vi "Loop_ACT_Drive.vi"() -> ()   [LabVIEW 2016, in "WC_Drive.lvlib"]
uses:
  WC_Drive.lvlib
  TypeDef/CLUSTER_Drive_HW_SRX_Status.ctl
  TypeDef/CLUSTER_4296_SRX_Status.ctl
  TypeDef/CLUSTER_SRX_Status Data.ctl
  TypeDef/CLUSTER_SRX_Encoder Data.ctl
  TypeDef/CLUSTER_SRX_PWM Data.ctl
  TypeDef/CLUSTER_SRX_Analog Data.ctl
  TypeDef/CLUSTER_SRX_Limit Switch Data.ctl
  TypeDef/CLUSTER_SRX_Profile Data.ctl
  TypeDef/ENUM_Drive_ACT Loop_Mode.ctl
  TypeDef/CLUSTER_Left and Right.ctl
  Globals/Global_STOP.vi
  Global_SM Write_Data Out.vi
  Global_ACT Write_Data Out.vi
panel:
  out "Right Data":dbl
  out "Left Data":dbl
  out "Cycle Time (S)":dbl format="%.3g"
  in  "Target Time(ms)":u32=50
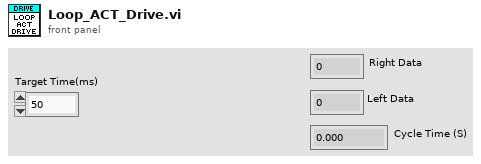
[diagram p1: front panel]
types:
  T1 = typedef "CLUSTER_Left and Right.ctl" = cluster{"Left":dbl, "Right":dbl}
  T2 = typedef "ENUM_Drive_ACT Loop_Mode.ctl" = enum16{"Stop", "VBus", "Profile"}
  T3 = typedef "CLUSTER_Drive_HW_SRX_Status.ctl" = cluster{"Rear Left":T4, "Rear Right":T4, "Front Left":T4, "Front Right":T4}
  T4 = typedef "CLUSTER_4296_SRX_Status.ctl" = cluster{"Status":T5, "Encoder":T6, "PWM ":T7, "Analog":T8, "Limit Switches":T9, "Profile":T10}
  T5 = typedef "CLUSTER_SRX_Status Data.ctl" = cluster{"Module Enabled":bool, "Current Profile Slot Select":dbl, "Brake is Enabled":bool, "Applied Throttle":dbl, "Current":dbl, "Battery Voltage":dbl, "Sticky Fault - Under Voltage":bool, "Temperature (C)":dbl, "Sticky Fault - Over Temp":bool, "CAN Error":errorcluster, "Control 5 Is Supported":bool}
  T6 = typedef "CLUSTER_SRX_Encoder Data.ctl" = cluster{"Closed Loop Error":dbl, "Sensor Position":dbl, "Sensor Velocity":dbl, "Encoder Position":dbl, "Encoder Velocity":dbl, "Encoder Index Count":dbl, "Encoder A Pin State":bool, "Encoder B Pin State":bool, "Encoder Index Pin State":bool, "Pos Div 8":bool, "Vel Div 4":bool}
  T7 = typedef "CLUSTER_SRX_PWM Data.ctl" = cluster{"Closed Loop Error":dbl, "Pulse Width Position":i32, "Pulse Width Velocity":i32, "Pulse Width Rise To Rise (us)":i32, "Pulse Width Rise To Fall (us)":i32}
  T8 = typedef "CLUSTER_SRX_Analog Data.ctl" = cluster{"Closed Loop Error":dbl, "Analog In":dbl, "Analog In Velocity":dbl}
  T9 = typedef "CLUSTER_SRX_Limit Switch Data.ctl" = cluster{"Forward Limit Switch Closed":bool, "Reverse Limit Switch Closed":bool, "Sticky Fault - Forward Limit":bool, "Sticky Fault - Reverse Limit":bool, "Sticky Fault - Forward Soft Limit":bool, "Sticky Fault - Reverse Soft Limit":bool}
  T10 = typedef "CLUSTER_SRX_Profile Data.ctl" = cluster{"Mot Prof Active Is Under Run":bool, "Mot Prof Active Has Under Run":bool, "Mot Prof Active Is Last":bool, "Mot Prof Active Velocity Only":bool, "Mot Prof Active Is Valid":bool, "Mot Prof Buffer Is Full":bool, "Mot Prof Active Profile Slot Select":i32, "Mot Prof NextID":i32, "Mot Prof Count":i32, "Mot Prof Active Velocity":dbl, "Mot Prof Active Position":dbl, "Mot Prof Output Enable":i32}
  T11 = typedef "WPI_RobotDriveDevRef.ctl" = cluster{"DevStatus":errorcluster, "Motors[]":T12[], "Square Inputs":bool, "Max Output":dbl}
  T12 = typedef "WPI_MotorControlDeviceRef.ctl" = cluster{"DeviceStatus":errorcluster, "Type":T13, "PWM":cluster{"PWM Channel":T14, "DeadBand":T15}, "CAN":cluster{"Device Number":u8, "SetOutput VI Ref":variant, "GetOutput VI Ref":variant, "Enable VI Ref":variant, "Disable VI Ref":variant, "Data":variant}, "Invert":bool}
  T13 = typedef "WPI_MotorControlType.ctl" = enum16{"PWM", "CAN"}
  T14 = typedef "FPGA_DIOPWMChannel.ctl" = enum8{"PWM 0", "PWM 1", "PWM 2", "PWM 3", "PWM 4", "PWM 5", "PWM 6", "PWM 7", "PWM 8", "PWM 9", "PWM MXP 0", "PWM MXP 1", "PWM MXP 2", "PWM MXP 3", "PWM MXP 4", "PWM MXP 5", "PWM MXP 6", "PWM MXP 7", "PWM MXP 8", "PWM MXP 9", "Invalid"}
  T15 = typedef "WPI_PWMDeadband.ctl" = cluster{"Name":string, "maxPositivePwm":i32, "minPositivePwm":i32, "centerPwm":i32, "maxNegativePwm":i32, "minNegativePwm":i32, "angularRange":u16}
  T16 = cluster{"RobotDriveDevRef":T11, "Target Time(ms)":u32, "Current Time":timestamp, "Previous Time":timestamp, "Cycle Time (S)":dbl, "SRX_Status":T3, "Mode":T2, "VBus":T1, "Cruise RPM":dbl, "MAX Velocity\n":dbl}
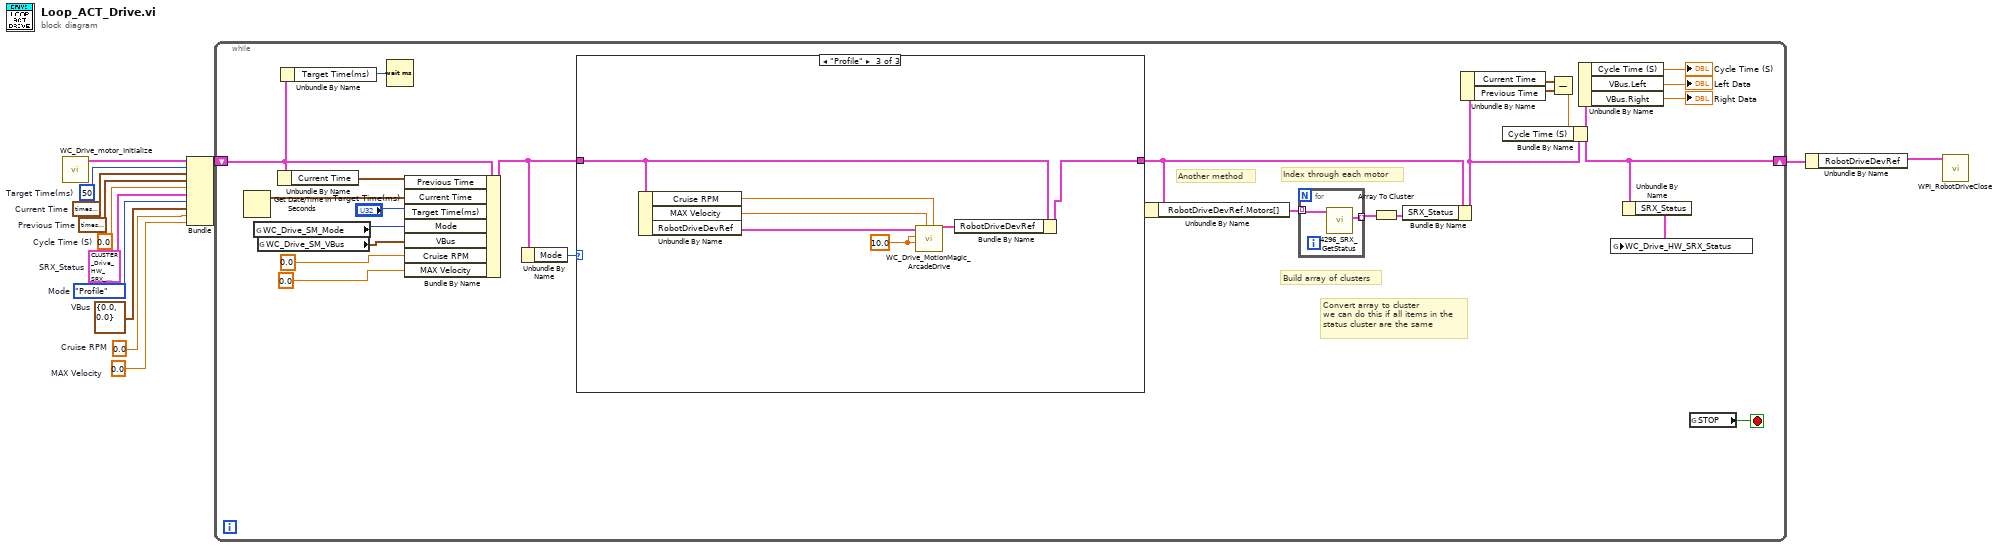
[diagram p0: block diagram]
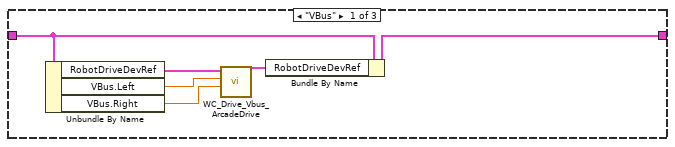
[diagram p2: hidden frame]
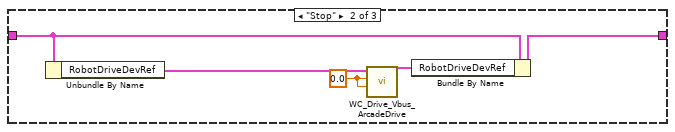
[diagram p3: hidden frame]
diagram:
  w1 = 0.0  # MAX Velocity
  w2 = 0.0  # Cruise RPM
  w3 = T1 {"Left"=0.0, "Right"=0.0}  # VBus
  w4 = ENUM_Drive_ACT_Loop_Mode."Profile"  # Mode
  w5 = T3 {"Rear Left"={"Status"={"Module Enabled"=FALSE, "Current Profile Slot Select"=0.0, "Brake is Enabled"=FALSE, "Applied Throttle"=0.0, "Current"=0.0, "Battery Voltage"=0.0, "Sticky Fault - Under Voltage"=FALSE, "Temperature (C)"=0.0, "Sticky Fault - Over Temp"=FALSE, "CAN Error"={"status"=FALSE, "code"=0, "source"=""}, "Control 5 Is Supported"=FALSE}, "Encoder"={"Closed Loop Error"=0.0, "Sensor Position"=0.0, "Sensor Velocity"=0.0, "Encoder Position"=0.0, "Encoder Velocity"=0.0, "Encoder Index Count"=0.0, "Encoder A Pin State"=FALSE, "Encoder B Pin State"=FALSE, "Encoder Index Pin State"=FALSE, "Pos Div 8"=FALSE, "Vel Div 4"=FALSE}, "PWM "={"Closed Loop Error"=0.0, "Pulse Width Position"=0, "Pulse Width Velocity"=0, "Pulse Width Rise To Rise (us)"=0, "Pulse Width Rise To Fall (us)"=0}, "Analog"={"Closed Loop Error"=0.0, "Analog In"=0.0, "Analog In Velocity"=0.0}, "Limit Switches"={"Forward Limit Switch Closed"=FALSE, "Reverse Limit Switch Closed"=FALSE, "Sticky Fault - Forward Limit"=FALSE, "Sticky Fault - Reverse Limit"=FALSE, "Sticky Fault - Forward Soft Limit"=FALSE, "Sticky Fault - Reverse Soft Limit"=FALSE}, "Profile"={"Mot Prof Active Is Under Run"=FALSE, "Mot Prof Active Has Under Run"=FALSE, "Mot Prof Active Is Last"=FALSE, "Mot Prof Active Velocity Only"=FALSE, "Mot Prof Active Is Valid"=FALSE, "Mot Prof Buffer Is Full"=FALSE, "Mot Prof Active Profile Slot Select"=0, "Mot Prof NextID"=0, "Mot Prof Count"=0, "Mot Prof Active Velocity"=0.0, "Mot Prof Active Position"=0.0, "Mot Prof Output Enable"=0}}, "Rear Right"={"Status"={"Module Enabled"=FALSE, "Current Profile Slot Select"=0.0, "Brake is Enabled"=FALSE, "Applied Throttle"=0.0, "Current"=0.0, "Battery Voltage"=0.0, "Sticky Fault - Under Voltage"=FALSE, "Temperature (C)"=0.0, "Sticky Fault - Over Temp"=FALSE, "CAN Error"={"status"=FALSE, "code"=0, "source"=""}, "Control 5 Is Supported"=FALSE}, "Encoder"={"Closed Loop Error"=0.0, "Sensor Position"=0.0, "Sensor Velocity"=0.0, "Encoder Position"=0.0, "Encoder Velocity"=0.0, "Encoder Index Count"=0.0, "Encoder A Pin State"=FALSE, "Encoder B Pin State"=FALSE, "Encoder Index Pin State"=FALSE, "Pos Div 8"=FALSE, "Vel Div 4"=FALSE}, "PWM "={"Closed Loop Error"=0.0, "Pulse Width Position"=0, "Pulse Width Velocity"=0, "Pulse Width Rise To Rise (us)"=0, "Pulse Width Rise To Fall (us)"=0}, "Analog"={"Closed Loop Error"=0.0, "Analog In"=0.0, "Analog In Velocity"=0.0}, "Limit Switches"={"Forward Limit Switch Closed"=FALSE, "Reverse Limit Switch Closed"=FALSE, "Sticky Fault - Forward Limit"=FALSE, "Sticky Fault - Reverse Limit"=FALSE, "Sticky Fault - Forward Soft Limit"=FALSE, "Sticky Fault - Reverse Soft Limit"=FALSE}, "Profile"={"Mot Prof Active Is Under Run"=FALSE, "Mot Prof Active Has Under Run"=FALSE, "Mot Prof Active Is Last"=FALSE, "Mot Prof Active Velocity Only"=FALSE, "Mot Prof Active Is Valid"=FALSE, "Mot Prof Buffer Is Full"=FALSE, "Mot Prof Active Profile Slot Select"=0, "Mot Prof NextID"=0, "Mot Prof Count"=0, "Mot Prof Active Velocity"=0.0, "Mot Prof Active Position"=0.0, "Mot Prof Output Enable"=0}}, "Front Left"={"Status"={"Module Enabled"=FALSE, "Current Profile Slot Select"=0.0, "Brake is Enabled"=FALSE, "Applied Throttle"=0.0, "Current"=0.0, "Battery Voltage"=0.0, "Sticky Fault - Under Voltage"=FALSE, "Temperature (C)"=0.0, "Sticky Fault - Over Temp"=FALSE, "CAN Error"={"status"=FALSE, "code"=0, "source"=""}, "Control 5 Is Supported"=FALSE}, "Encoder"={"Closed Loop Error"=0.0, "Sensor Position"=0.0, "Sensor Velocity"=0.0, "Encoder Position"=0.0, "Encoder Velocity"=0.0, "Encoder Index Count"=0.0, "Encoder A Pin State"=FALSE, "Encoder B Pin State"=FALSE, "Encoder Index Pin State"=FALSE, "Pos Div 8"=FALSE, "Vel Div 4"=FALSE}, "PWM "={"Closed Loop Error"=0.0, "Pulse Width Position"=0, "Pulse Width Velocity"=0, "Pulse Width Rise To Rise (us)"=0, "Pulse Width Rise To Fall (us)"=0}, "Analog"={"Closed Loop Error"=0.0, "Analog In"=0.0, "Analog In Velocity"=0.0}, "Limit Switches"={"Forward Limit Switch Closed"=FALSE, "Reverse Limit Switch Closed"=FALSE, "Sticky Fault - Forward Limit"=FALSE, "Sticky Fault - Reverse Limit"=FALSE, "Sticky Fault - Forward Soft Limit"=FALSE, "Sticky Fault - Reverse Soft Limit"=FALSE}, "Profile"={"Mot Prof Active Is Under Run"=FALSE, "Mot Prof Active Has Under Run"=FALSE, "Mot Prof Active Is Last"=FALSE, "Mot Prof Active Velocity Only"=FALSE, "Mot Prof Active Is Valid"=FALSE, "Mot Prof Buffer Is Full"=FALSE, "Mot Prof Active Profile Slot Select"=0, "Mot Prof NextID"=0, "Mot Prof Count"=0, "Mot Prof Active Velocity"=0.0, "Mot Prof Active Position"=0.0, "Mot Prof Output Enable"=0}}, "Front Right"={"Status"={"Module Enabled"=FALSE, "Current Profile Slot Select"=0.0, "Brake is Enabled"=FALSE, "Applied Throttle"=0.0, "Current"=0.0, "Battery Voltage"=0.0, "Sticky Fault - Under Voltage"=FALSE, "Temperature (C)"=0.0, "Sticky Fault - Over Temp"=FALSE, "CAN Error"={"status"=FALSE, "code"=0, "source"=""}, "Control 5 Is Supported"=FALSE}, "Encoder"={"Closed Loop Error"=0.0, "Sensor Position"=0.0, "Sensor Velocity"=0.0, "Encoder Position"=0.0, "Encoder Velocity"=0.0, "Encoder Index Count"=0.0, "Encoder A Pin State"=FALSE, "Encoder B Pin State"=FALSE, "Encoder Index Pin State"=FALSE, "Pos Div 8"=FALSE, "Vel Div 4"=FALSE}, "PWM "={"Closed Loop Error"=0.0, "Pulse Width Position"=0, "Pulse Width Velocity"=0, "Pulse Width Rise To Rise (us)"=0, "Pulse Width Rise To Fall (us)"=0}, "Analog"={"Closed Loop Error"=0.0, "Analog In"=0.0, "Analog In Velocity"=0.0}, "Limit Switches"={"Forward Limit Switch Closed"=FALSE, "Reverse Limit Switch Closed"=FALSE, "Sticky Fault - Forward Limit"=FALSE, "Sticky Fault - Reverse Limit"=FALSE, "Sticky Fault - Forward Soft Limit"=FALSE, "Sticky Fault - Reverse Soft Limit"=FALSE}, "Profile"={"Mot Prof Active Is Under Run"=FALSE, "Mot Prof Active Has Under Run"=FALSE, "Mot Prof Active Is Last"=FALSE, "Mot Prof Active Velocity Only"=FALSE, "Mot Prof Active Is Valid"=FALSE, "Mot Prof Buffer Is Full"=FALSE, "Mot Prof Active Profile Slot Select"=0, "Mot Prof NextID"=0, "Mot Prof Count"=0, "Mot Prof Active Velocity"=0.0, "Mot Prof Active Position"=0.0, "Mot Prof Output Enable"=0}}}  # SRX_Status
  w8 = 0.0  # Cycle Time (S)
  w13 = timestamp(0 s since 1904-01-01)  # Previous Time
  w12 = timestamp(0 s since 1904-01-01)  # Current Time
  w11 = u32 50  # Target Time(ms)
  n1 = call "WC_Drive_motor_Initialize.vi"() -> ("RobotDriveDevRef"=w7:T11)  [unwired: 11 in]
  n2 = Bundle("RobotDriveDevRef"=w7, "Target Time(ms)"=w11, "Current Time"=w12, "Previous Time"=w13, "Cycle Time (S)"=w8, "SRX_Status"=w5, "Mode"=w4, "VBus"=w3, "Cruise RPM"=w2, "MAX Velocity"=w1) -> (w10:T16)  [unwired: 1 in]
  n3 = while {
    shift-right: [w23] -> w9
    shift-left: w10 -> [w20]
    stop <- w38 stop-if-true
    # "Build array of clusters"
    # "Convert array to cluster\nwe can do this if all items in the\nstatus cluster are the same"
    # "Index through each motor"
    # "Another method"
    n4 = Get Date/Time In Seconds() -> (seconds since 1Jan1904=w37:timestamp)
    n5 = global read "Global_SM Write_Data Out.vi" "WC_Drive_SM_Mode"() -> (w27:T2)
    n6 = global read "Global_SM Write_Data Out.vi" "WC_Drive_SM_VBus"() -> (w16:T1)
    n7 = Unbundle By Name(w20) -> ("Current Time"=w36:timestamp)
    n8 = Unbundle By Name(w20) -> ("Target Time(ms)"=w32:u32)
    n9 = Wait (ms)(milliseconds to wait=w32) -> ()  [unwired: 1 out]
    n10 = Bundle By Name(cluster=w20, "Previous Time"=w36, "Current Time"=w37, "Target Time(ms)"="Target Time(ms)", "Mode"=w27, "VBus"=w16, "Cruise RPM"=0.0, "MAX Velocity"=0.0) -> (w26:T16)
    n11 = Unbundle By Name(w26) -> ("Mode"=w25:T2)
    n12 = case shown="\"Profile\"" w25 {
      tunnel: w26 -> [w42 w50 w54]
      tunnel: [w41 w49 w55] -> w21
      frame "VBus" {
        n13 = Unbundle By Name(w42) -> ("RobotDriveDevRef"=w46:T11, "VBus.Left"=w45:dbl, "VBus.Right"=w44:dbl)
        n14 = call "WC_Drive_Vbus_ArcadeDrive.vi"("Right Value"=w44, "Left Value"=w45, "RobotDriveDevRef"=w46) -> ("RobotDriveDevRef Out"=w43:T11)  [unwired: 7 in, 1 out]
        n15 = Bundle By Name(cluster=w42, "RobotDriveDevRef"=w43) -> (w41:T16)
      }
      frame "Stop" {
        w48 = 0.0 ("X axis value")
        n16 = Unbundle By Name(w50) -> ("RobotDriveDevRef"=w47:T11)
        n17 = call "WC_Drive_Vbus_ArcadeDrive.vi"("Right Value"=w48, "Left Value"=w48, "RobotDriveDevRef"=w47) -> ("RobotDriveDevRef Out"=w51:T11)  [unwired: 7 in, 1 out]
        n18 = Bundle By Name(cluster=w50, "RobotDriveDevRef"=w51) -> (w49:T16)
      }
      frame "Profile" {
        w57 = 10.0 ("X axis value")
        n19 = Unbundle By Name(w54) -> ("Cruise RPM"=w53:dbl, "MAX Velocity"=w52:dbl, "RobotDriveDevRef"=w58:T11)
        n20 = call "WC_Drive_MotionMagic_ArcadeDrive.vi"("Cruise RPM"=w53, "Max Velocity"=w52, "Right Value"=w57, "Left Value"=w57, "RobotDriveDevRef"=w58) -> ("RobotDriveDevRef Out"=w56:T11)  [unwired: 5 in, 1 out]
        n21 = Bundle By Name(cluster=w54, "RobotDriveDevRef"=w56) -> (w55:T16)
      }
    }
    n22 = Unbundle By Name(w21) -> ("RobotDriveDevRef.Motors[]"=w19:T12[])
    n23 = for {
      tunnel: w19 -> [w40] mode=indexing
      tunnel: [w39] -> w18 mode=indexing
      n24 = call "4296_SRX_GetStatus.vi"("CAN Talon SRX Ref"=w40) -> ("4296 SRX Status Out"=w39:T4)  [unwired: 8 in, 2 out]
    }
    n25 = Array To Cluster(array=w18) -> (cluster=w17:cluster{"[0]":T4, "[1]":T4, "[2]":T4, "[3]":T4})
    n26 = Bundle By Name(cluster=w21, "SRX_Status"=w17) -> (w22:T16)
    n27 = Unbundle By Name(w22) -> ("Current Time"=w35:timestamp, "Previous Time"=w34:timestamp)
    n28 = Subtract(x=w35, y=w34) -> (x-y=w24:dbl)
    n29 = Bundle By Name(cluster=w22, "Cycle Time (S)"=w24) -> (w23:T16)
    n30 = Unbundle By Name(w23) -> ("Cycle Time (S)"=→"Cycle Time (S)":dbl, "VBus.Left"=→"Left Data":dbl, "VBus.Right"=→"Right Data":dbl)
    n31 = Unbundle By Name(w23) -> ("SRX_Status"=w28:T3)
    n32 = global write "Global_ACT Write_Data Out.vi" "WC_Drive_HW_SRX_Status"(w28) -> ()
    n33 = global read "Global_STOP.vi" "STOP"() -> (w38:bool)
  }
  n34 = Unbundle By Name(w9) -> ("RobotDriveDevRef"=w6:T11)
  n35 = call <vilib>:"WPI_RobotDriveClose.vi"("RobotDriveDevRef"=w6) -> ()  [unwired: 10 in, 1 out]
